vi "Build Sequence.vi"(6 "Options":string[](array[string]), 11 "Car Wash Model in":refnum<class "Car Wash Model.lvclass">) -> (3 "Car Wash Model out":refnum<class "Car Wash Model.lvclass">, 4 "Sequence":string[](array[string]))   [LabVIEW 2019, in "Car Wash Model.lvclass"]
uses:
  <vilib>/gpm_packages/@cs/Car-wash/Source/Car Wash Model/Car Wash Model/Car Wash Model.lvclass
  <vilib>/gpm_packages/@cs/Car-wash/Source/Car Wash Model/Car Wash Model/Car Wash Model.lvclass/Car Wash Model.ctl
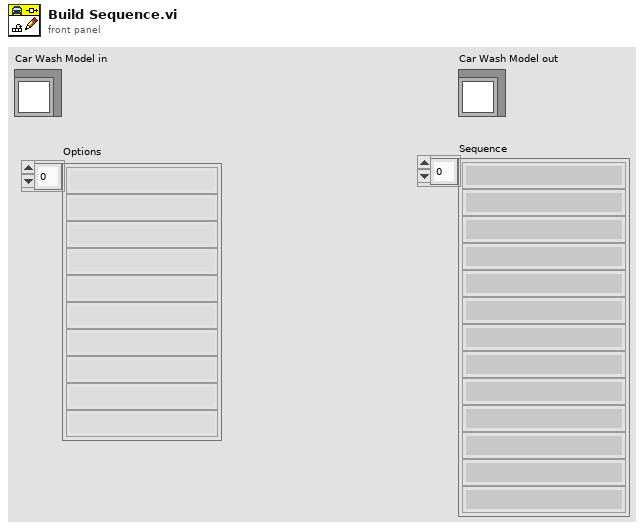
[diagram p1: front panel]
types:
  T1 = typedef "Option Definition.ctl" = cluster{"Name":string, "Time (mSec)":i32, "Station":u8}
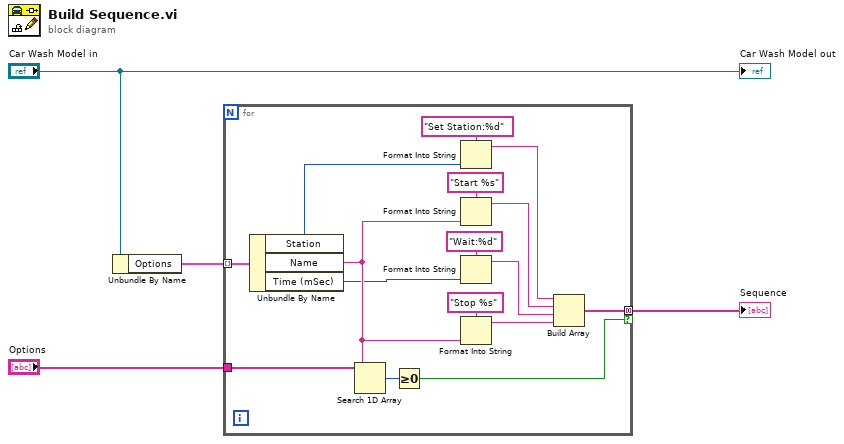
[diagram p0: block diagram]
diagram:
  n1 = Unbundle By Name("Car Wash Model in") -> ("Options"=w2:T1[])
  n2 = for {
    tunnel: w2 -> [w19] mode=indexing
    tunnel: "Options" -> [w20]
    tunnel: [w6] -> w1 mode=concatenating if=w5
    n3 = Unbundle By Name(w19) -> ("Station"=w11:u8, "Name"=w15:string, "Time (mSec)"=w13:i32)
    n4 = Search 1D Array(1D array=w20, element=w15) -> (index of element=w18:i32)  [unwired: 1 in]
    n5 = Greater Or Equal To 0?(x=w18) -> (x >= 0?=w5:bool)
    n6 = Format Into String(format string="Set Station:%d", w11) -> (resulting string=w10:string)  [unwired: 2 in, 1 out]
    n7 = Format Into String(format string="Start %s", w15) -> (resulting string=w9:string)  [unwired: 2 in, 1 out]
    n8 = Format Into String(format string="Wait:%d", w13) -> (resulting string=w8:string)  [unwired: 2 in, 1 out]
    n9 = Format Into String(format string="Stop %s", w15) -> (resulting string=w7:string)  [unwired: 2 in, 1 out]
    n10 = Build Array(w10, w9, w8, w7) -> (w6:string[])
  }
  "Sequence" <- w1
  "Car Wash Model out" <- "Car Wash Model in"
